vi "GetStrArrFromLIstBox.vi"(11 "ArrayRef in":refnum<vi>) -> (2 "result":string[](array[string]), 3 "ArrayRef out":refnum<vi>)   [LabVIEW 2018, in "Library-Ctrl.lvlib"]
uses:
  Library-Ctrl.lvlib
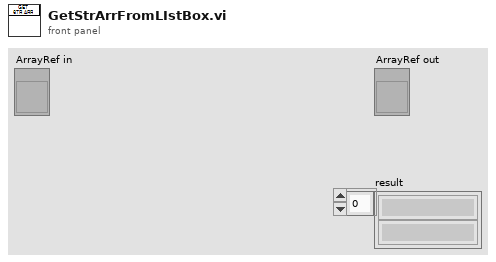
[diagram p1: front panel]
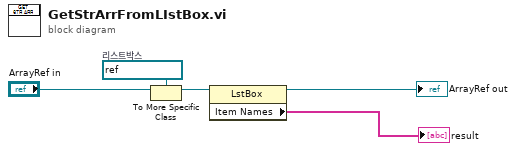
[diagram p0: block diagram]
diagram:
  w4 = refnum<vi> refnum  # 리스트박스
  n1 = To More Specific Class(target class=w4, reference="ArrayRef in") -> (specific class reference=w2:refnum<vi>)  [unwired: 1 in, 1 out]
  n2 = property class="LstBox"(reference=w2) -> (reference out=→"ArrayRef out":refnum<vi>, "Item Names"=→"result":string[])  [unwired: 1 in, 1 out]
